vi "save.series.vi"(8 "error in":errorcluster, 11 "data":T1) -> (0 "error out":errorcluster)   [LabVIEW 2024]
uses:
  series.reply.ctl
  <vilib>/addons/_JKI.lib/Serialization/JSON/JKI JSON Serialization.lvlib
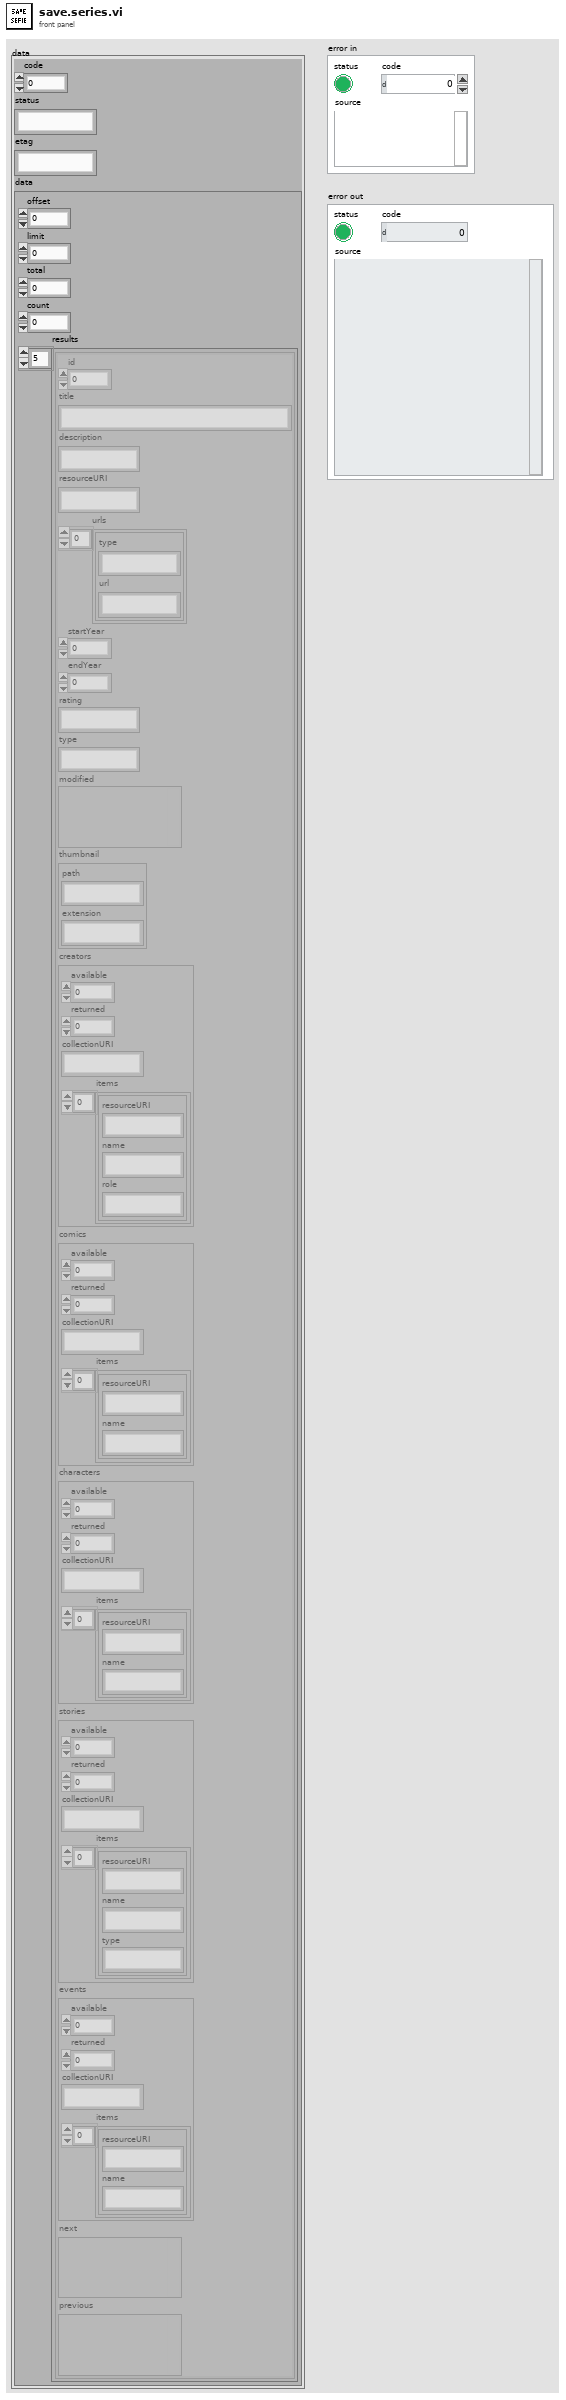
[diagram p1: front panel]
types:
  T1 = typedef "series.reply.ctl" = cluster{"code":i32, "status":string, "etag":string, "data":cluster{"offset":i32, "limit":i32, "total":i32, "count":i32, "results":cluster{"id":i32, "title":string, "description":string, "resourceURI":string, "urls":cluster{"type":string, "url":string}[], "startYear":i32, "endYear":i32, "rating":string, "type":string, "modified":variant, "thumbnail":cluster{"path":string, "extension":string}, "creators":cluster{"available":i32, "returned":i32, "collectionURI":string, "items":cluster{"resourceURI":string, "name":string, "role":string}[]}, "comics":cluster{"available":i32, "returned":i32, "collectionURI":string, "items":cluster{"resourceURI":string, "name":string}[]}, "characters":cluster{"available":i32, "returned":i32, "collectionURI":string, "items":cluster{"resourceURI":string, "name":string}[]}, "stories":cluster{"available":i32, "returned":i32, "collectionURI":string, "items":cluster{"resourceURI":string, "name":string, "type":string}[]}, "events":cluster{"available":i32, "returned":i32, "collectionURI":string, "items":cluster{"resourceURI":string, "name":string}[]}, "next":variant, "previous":variant}[]}}
  T2 = enum16{"open", "replace", "create", "open or create", "replace or create", "replace or create with confirmation"}
  T3 = cluster{"id":i32, "title":string, "description":string, "resourceURI":string, "urls":cluster{"type":string, "url":string}[], "startYear":i32, "endYear":i32, "rating":string, "type":string, "modified":variant, "thumbnail":cluster{"path":string, "extension":string}, "creators":cluster{"available":i32, "returned":i32, "collectionURI":string, "items":cluster{"resourceURI":string, "name":string, "role":string}[]}, "comics":cluster{"available":i32, "returned":i32, "collectionURI":string, "items":cluster{"resourceURI":string, "name":string}[]}, "characters":cluster{"available":i32, "returned":i32, "collectionURI":string, "items":cluster{"resourceURI":string, "name":string}[]}, "stories":cluster{"available":i32, "returned":i32, "collectionURI":string, "items":cluster{"resourceURI":string, "name":string, "type":string}[]}, "events":cluster{"available":i32, "returned":i32, "collectionURI":string, "items":cluster{"resourceURI":string, "name":string}[]}, "next":variant, "previous":variant}[]
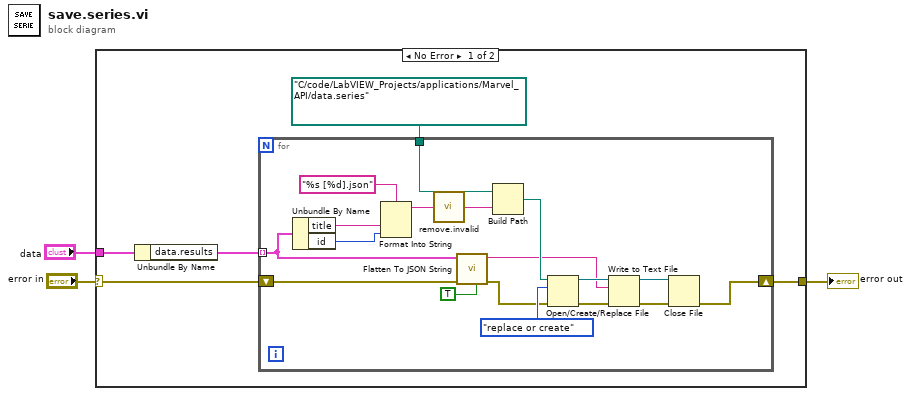
[diagram p0: block diagram]
diagram:
  n1 = case shown="No Error" "error in" {
    selector: "error in" -> [w4 w27]
    tunnel: "data" -> [w8 _]
    tunnel: [w5 w27] -> w2
    frame No Error {
      n2 = Unbundle By Name(w8) -> ("data.results"=w7:T3)
      n3 = for {
        tunnel: w7 -> [w16] mode=indexing
        tunnel: path "C:/code/LabVIEW_Projects/applications/Marvel_API/data.series" ("file (use dialog)") -> [w24]
        shift-right: [w17] -> w5
        shift-left: w4 -> [w14]
        n4 = Unbundle By Name(w16) -> ("title"=w10:string, "id"=w9:i32)
        n5 = Format Into String(format string="%s [%d].json", w10, w9) -> (resulting string=w25:string)  [unwired: 2 in, 1 out]
        n6 = call "remove.invalid.vi"("string in"=w25) -> ("string out"=w11:string)
        n7 = call <vilib>:"Flatten To JSON String.vi"("Enums As String (F)"=TRUE, "error in"=w14, "Variant"=w16) -> ("error out"=w13:errorcluster, "JSON String"=w15:string)  [unwired: 7 in]
        n8 = Build Path(base path=w24, name or relative path=w11) -> (appended path=w23:path)
        n9 = Open/Create/Replace File(file path (use dialog)=w23, error in=w13, operation (0:open)=T2."replace or create") -> (refnum out=w21:refnum<file>, error out=w20:errorcluster)  [unwired: 3 in, 1 out]
        n10 = Write to Text File(file (use dialog)=w21, text=w15, error in=w20) -> (refnum out=w18:refnum<file>, error out=w19:errorcluster)  [unwired: 1 in, 1 out]
        n11 = Close File(refnum=w18, error in=w19) -> (error out=w17:errorcluster)  [unwired: 1 out]
      }
    }
    frame Error {
    }
  }
  "error out" <- w2
